vi "Draw Diamond.vi"(6 "Draw Para":T2={"fill?(F)"=TRUE, "color(black)"=0, "pen"={"Width"=1, "Style"=enum."Solid"}}, 8 "错误输入":errorcluster, 9 "Offset":T1, 10 "Center":T1, 11 "Pic in":picture) -> (0 "错误输出":errorcluster, 3 "Pic out":picture)   [LabVIEW 2012, in "Picture Box Tools.lvlib" / "Basic Shape.lvlib"]
uses:
  Basic Shape.lvlib
  Point Custom Control.ctl
  Draw Para Custom Control.ctl
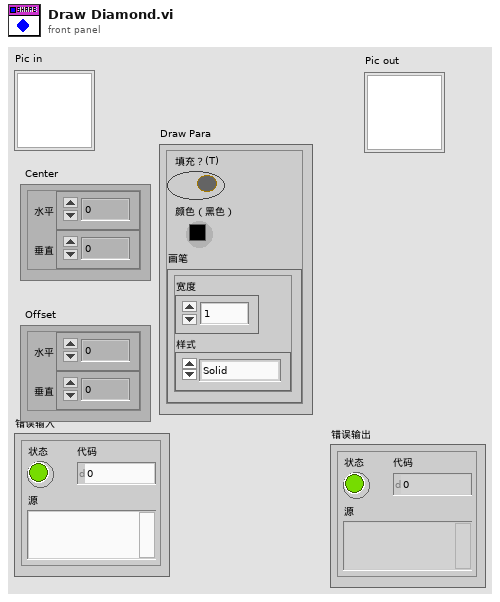
[diagram p1: front panel]
types:
  T1 = typedef "Picture Box Tools.lvlib/Basic Shape.lvlib/Point Custom Control.ctl" = cluster{"horizontal":i16, "vertical":i16}
  T2 = typedef "Picture Box Tools.lvlib/Basic Shape.lvlib/Draw Para Custom Control.ctl" = cluster{"fill?(F)":bool, "color(black)":u32, "pen":cluster{"Width":u16, "Style":enum32{"Solid", "Dash", "Dot", "DashDot", "DashDotDot"}}}
  T3 = cluster{"Width":u16, "Style":enum32{"Solid", "Dash", "Dot", "DashDot", "DashDotDot"}}
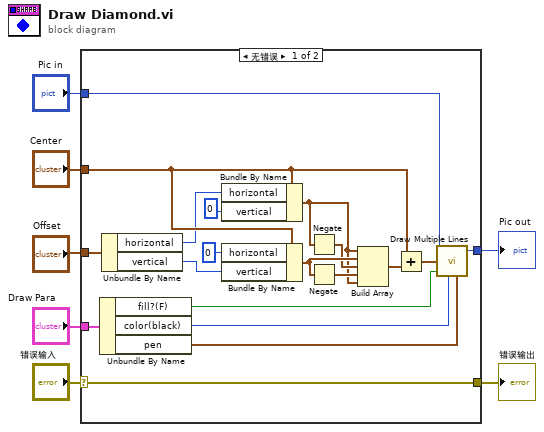
[diagram p0: block diagram]
diagram:
  n1 = case shown="无错误" "错误输入" {
    selector: "错误输入" -> [w15 w28]
    tunnel: [w15 w28] -> w6
    tunnel: "Pic in" -> [w14 w27]
    tunnel: "Center" -> [w13 _]
    tunnel: "Draw Para" -> [w12 _]
    tunnel: [w11 w27] -> w2
    tunnel: "Offset" -> [w10 _]
    frame No Error {
      n2 = Unbundle By Name(w12) -> ("fill?(F)"=w18:bool, "color(black)"=w17:u32, "pen"=w16:T3)
      n3 = Unbundle By Name(w10) -> ("horizontal"=w9:i16, "vertical"=w8:i16)
      n4 = Bundle By Name(cluster=w13, "horizontal"=w9, "vertical"=i16 0) -> (w19:T1)
      n5 = Bundle By Name(cluster=w13, "horizontal"=i16 0, "vertical"=w8) -> (w24:T1)
      n6 = Negate(x=w19) -> (-x=w23:T1)
      n7 = Negate(x=w24) -> (-x=w22:T1)
      n8 = Build Array(w19, w24, w23, w22, w19) -> (w21:T1[])
      n9 = Add(x=w13, y=w21) -> (x+y=w20:T1[])
      n10 = call <vilib>:"Draw Multiple Lines.vi"("picture"=w14, "line endpoints"=w20, "fill?(F)"=w18, "color(black)"=w17, "pen"=w16) -> ("new picture"=w11:picture)  [unwired: 4 in]
    }
    frame Error {
    }
  }
  "错误输出" <- w6
  "Pic out" <- w2
